vi "Sud_bound_freq_differential.vi"(8 "Slop factor":dbl=1.0, 9 "Max delta freq":dbl, 10 "Prior Frequency estimate":dbl, 11 "Next Frequency estimate":dbl) -> (2 "Slop factor (feedback)":dbl=1.0, 3 "Next Frequency estimate (Bounded)":dbl)   [LabVIEW 2021]
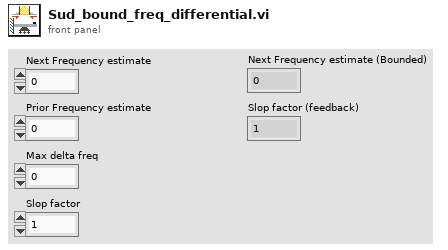
[diagram p1: front panel]
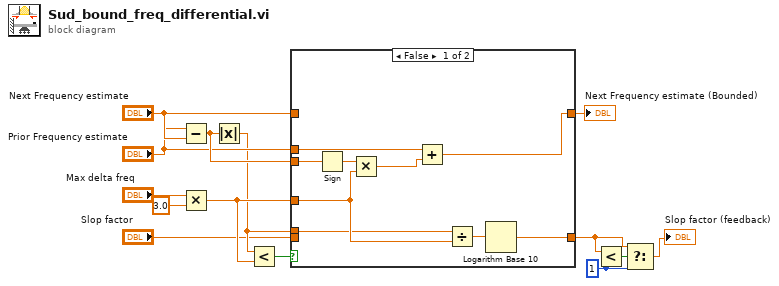
[diagram p0: block diagram]
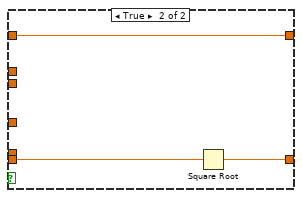
[diagram p2: hidden frame]
diagram:
  w2 = 1
  n1 = Subtract(x="Prior Frequency estimate", y="Next Frequency estimate") -> (x-y=w12:dbl)
  n2 = Multiply(x="Max delta freq", y=3.0) -> (x*y=w11:dbl)
  n3 = Absolute Value(x=w12) -> (abs(x)=w7:dbl)
  n4 = Less?(x=w7, y=w11) -> (x < y?=w13:bool)
  n5 = case shown="False" w13 {
    tunnel: "Next Frequency estimate" -> [_ w26]
    tunnel: [w19 w26] -> w10
    tunnel: "Prior Frequency estimate" -> [w20 _]
    tunnel: w12 -> [w23 _]
    tunnel: w11 -> [w17 _]
    tunnel: [w15 w25] -> w4
    tunnel: w7 -> [w16 _]
    tunnel: "Slop factor" -> [_ w24]
    frame False {
      n6 = Sign(1:w23) -> (0:w22:dbl)
      n7 = Multiply(x=w22, y=w17) -> (x*y=w21:dbl)
      n8 = Add(x=w20, y=w21) -> (x+y=w19:dbl)
      n9 = Divide(x=w16, y=w17) -> (x/y=w18:dbl)
      n10 = Logarithm Base 10(1:w18) -> (0:w15:dbl)
    }
    frame True {
      n11 = Square Root(x=w24) -> (sqrt(x)=w25:dbl)
    }
  }
  "Next Frequency estimate (Bounded)" <- w10
  n12 = Less?(x=w4, y=w2) -> (x < y?=w5:bool)
  n13 = Select(t=w4, s=w5, f=w2) -> (s? t:f=→"Slop factor (feedback)":dbl)
